vi "Temperature Converter.vi"() -> ()   [LabVIEW 2023]
panel:
  out "Temperature (C)":string
  out "Temperature (F)":string
  out "Waveform Graph":dbl[](graph)
  in  "stop":bool
  out "Waveform Chart":dbl(graph)
  in  "Boolean":bool
  out "Thermometer (F)":dbl(slide) scale=0.0..200.0
  in  "Temperaturee (C)":dbl(slide) scale=0.0..100.0
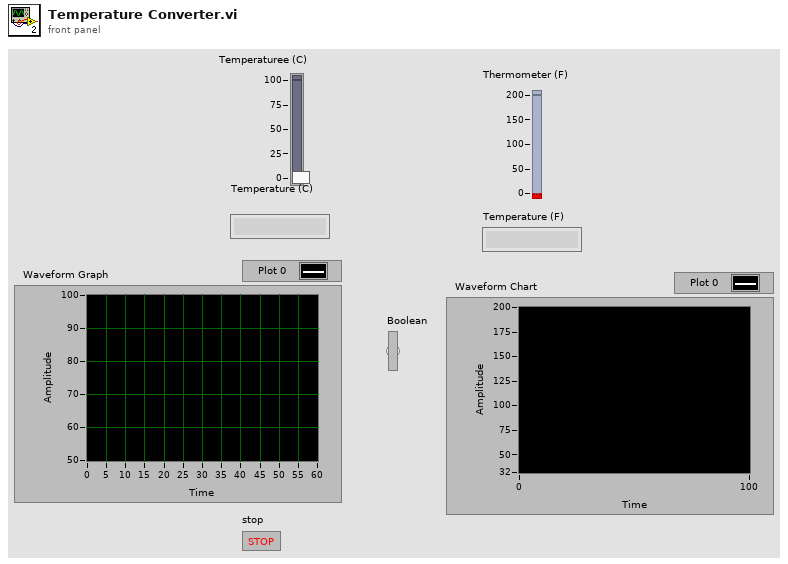
[diagram p1: front panel]
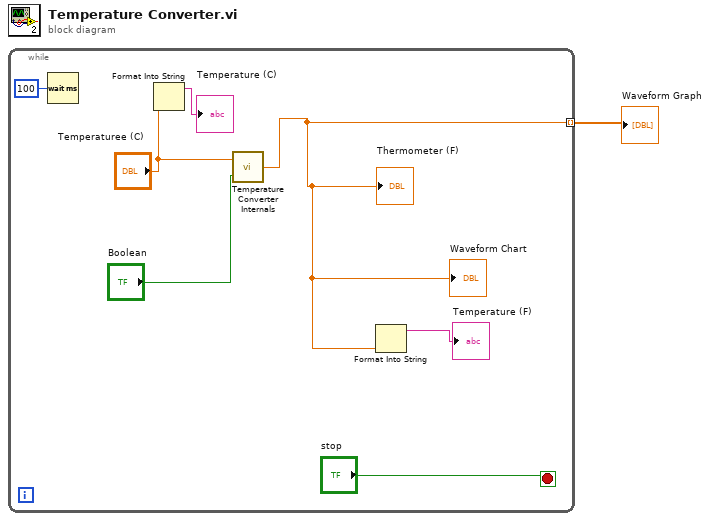
[diagram p0: block diagram]
diagram:
  n1 = while {
    tunnel: [w3] -> w1 mode=indexing
    stop <- "stop" stop-if-true
    n2 = Wait (ms)(milliseconds to wait=u32 100) -> ()  [unwired: 1 out]
    n3 = Format Into String("Temperaturee (C)") -> (resulting string=→"Temperature (C)":string)  [unwired: 3 in, 1 out]
    n4 = call "Temperature Converter Internals.vi"("Boolean"="Boolean", "Temperaturee (C)"="Temperaturee (C)") -> ("Numeric"=w3:dbl)
    "Thermometer (F)" <- w3
    "Waveform Chart" <- w3
    n5 = Format Into String(w3) -> (resulting string=→"Temperature (F)":string)  [unwired: 3 in, 1 out]
  }
  "Waveform Graph" <- w1
